vi "graph problems 2.vi"() -> ()   [LabVIEW 2018]
uses:
  <vilib>/DAQmx/configure/timing.llb/DAQmx Timing (Sample Clock).vi
  <vilib>/DAQmx/read.llb/DAQmx Read (Analog Wfm 1Chan NSamp).vi
  <vilib>/DAQmx/create/channels.llb/DAQmx Create Channel (AO-Voltage-Basic).vi
  <vilib>/DAQmx/write.llb/DAQmx Write (Analog DBL 1Chan 1Samp).vi
  <vilib>/DAQmx/create/channels.llb/DAQmx Create Channel (AI-Voltage-Basic).vi
panel:
  out "Waveform Graph":waveform(dbl)(graph)
  in  "physical channels 2":tag
  in  "stop":bool
  in  "physical channels":tag
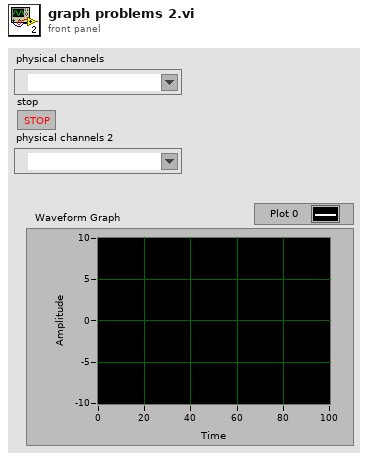
[diagram p1: front panel]
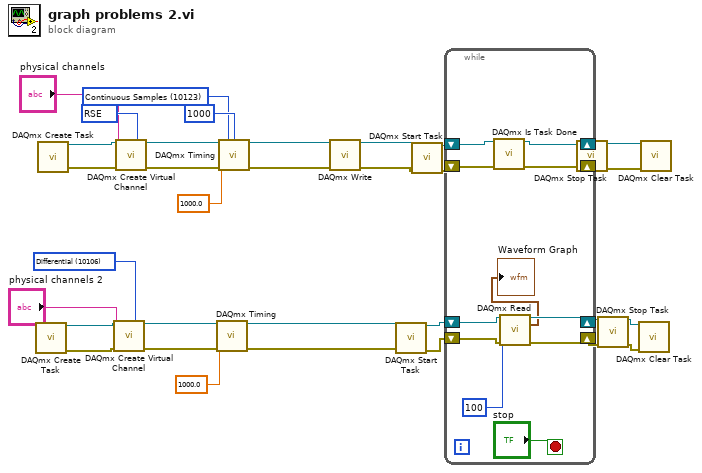
[diagram p0: block diagram]
diagram:
  w6 = 10106 items=["Default"=-1, "RSE"=10083, "NRSE"=10078, "Differential"=10106, "Pseudodifferential"=12529] ("input terminal configuration")
  w14 = 10123 items=["Finite Samples"=10178, "Continuous Samples"=10123, "Hardware Timed Single Point"=12522] ("sample mode")
  w30 = 10083 items=["Default"=-1, "RSE"=10083, "Differential"=10106, "Pseudodifferential"=12529] ("output terminal configuration")
  n1 = call <vilib>:"DAQmx Create Task.vi"() -> ("task out"=w13:refnum<k21>, "error out"=w10:errorcluster)  [unwired: 14 in]
  n2 = call <vilib>:"DAQmx Create Task.vi"() -> ("task out"=w29:refnum<k21>, "error out"=w23:errorcluster)  [unwired: 14 in]
  n3 = call-poly <vilib>:"DAQmx Create Virtual Channel.vi"("task in"=w13, "input terminal configuration"=w6, "physical channels"="physical channels 2", "error in"=w10) -> ("task out"=w12:refnum<k21>, "error out"=w9:errorcluster)  [unwired: 10 in]
  n4 = call-poly <vilib>:"DAQmx Create Virtual Channel.vi"("task in"=w29, "output terminal configuration"=w30, "physical channels"="physical channels", "error in"=w23) -> ("task out"=w28:refnum<k21>, "error out"=w22:errorcluster)  [unwired: 10 in]
  n5 = call-poly <vilib>:"DAQmx Timing.vi"("task/channels in"=w12, "rate"=1000.0, "error in"=w9) -> ("task out"=w11:refnum<k21>, "error out"=w8:errorcluster)  [unwired: 11 in]
  n6 = call-poly <vilib>:"DAQmx Timing.vi"("task/channels in"=w28, "sample mode"=w14, "samples per channel"=1000, "rate"=1000.0, "error in"=w22) -> ("task out"=w27:refnum<k21>, "error out"=w21:errorcluster)  [unwired: 9 in]
  n7 = call-poly <vilib>:"DAQmx Write.vi"("task/channels in"=w27, "error in"=w21) -> ("task out"=w26:refnum<k21>, "error out"=w20:errorcluster)  [unwired: 11 in, 1 out]
  n8 = call <vilib>:"DAQmx Start Task.vi"("task/channels in"=w11, "error in"=w8) -> ("task out"=w4:refnum<k21>, "error out"=w2:errorcluster)  [unwired: 12 in]
  n9 = call <vilib>:"DAQmx Start Task.vi"("task/channels in"=w26, "error in"=w20) -> ("task out"=w25:refnum<k21>, "error out"=w19:errorcluster)  [unwired: 12 in]
  n10 = while {
    shift-right: [w44] -> w24
    shift-left: w25 -> [w45]
    shift-right: [w42] -> w18
    shift-left: w19 -> [w43]
    shift-right: [w39] -> w3
    shift-left: w4 -> [w40]
    shift-right: [w38] -> w1
    shift-left: w2 -> [w37]
    stop <- "stop" stop-if-true
    n11 = call <vilib>:"DAQmx Is Task Done.vi"("task/channels in"=w45, "error in"=w43) -> ("task out"=w44:refnum<k21>, "error out"=w42:errorcluster)  [unwired: 11 in, 1 out]
    n12 = call-poly <vilib>:"DAQmx Read.vi"("task/channels in"=w40, "number of samples per channel"=100, "error in"=w37) -> ("task out"=w39:refnum<k21>, "data"=→"Waveform Graph":waveform(dbl), "error out"=w38:errorcluster)  [unwired: 10 in]
  }
  n13 = call <vilib>:"DAQmx Stop Task.vi"("task/channels in"=w24, "error in"=w18) -> ("task out"=w34:refnum<k21>, "error out"=w33:errorcluster)  [unwired: 12 in]
  n14 = call <vilib>:"DAQmx Stop Task.vi"("task/channels in"=w3, "error in"=w1) -> ("task out"=w31:refnum<k21>, "error out"=w32:errorcluster)  [unwired: 12 in]
  n15 = call <vilib>:"DAQmx Clear Task.vi"("task in"=w31, "error in"=w32) -> ()  [unwired: 13 in, 1 out]
  n16 = call <vilib>:"DAQmx Clear Task.vi"("task in"=w34, "error in"=w33) -> ()  [unwired: 13 in, 1 out]
